vi "Configure Current Limit.vi"(7 "Behavior (0: Regulate)":u16(ring) items=["Regulate", "Trip"], 8 "error in (no error)":errorcluster, 9 "Current Limit (0.0 A)":dbl format="%.3g", 10 "Channel (1: Channel 1)":i32(ring)=1 items=["Channel 1"=1, "Channel 2"=2, "Channel 3"=3], 11 "VISA resource name":refnum<visa-resource-name>) -> (0 "error out":errorcluster, 3 "VISA resource name out":refnum<visa-resource-name>)   [LabVIEW 2020, in "Agilent E363X Series.lvlib"]
doc: "Configures the current limit. Specify the output current limit value and the behavior of the power supply when the output current is greater than or equal to that value."
uses:
  Agilent E363X Series.lvlib
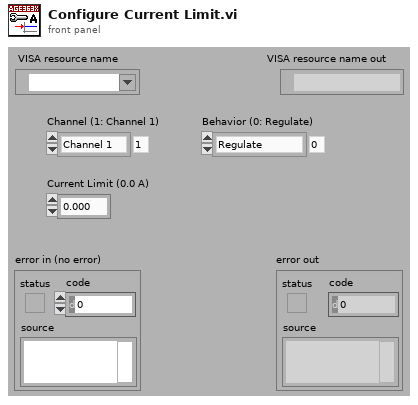
[diagram p1: front panel]
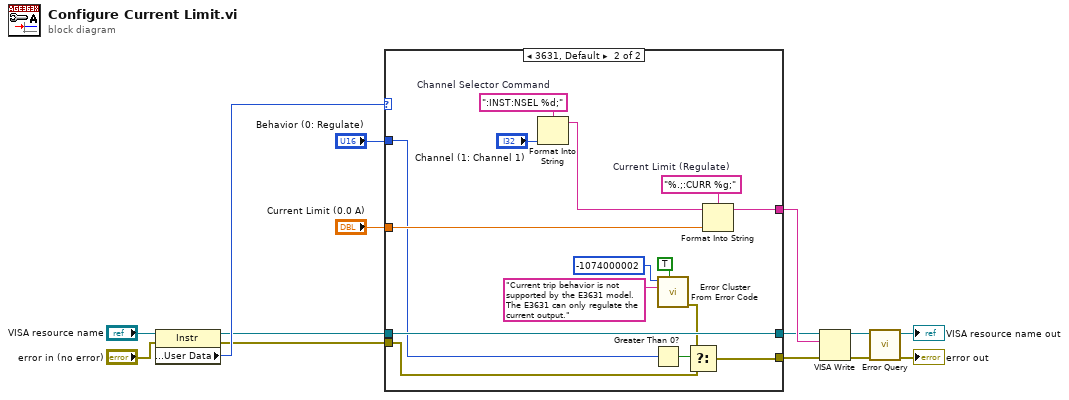
[diagram p0: block diagram]
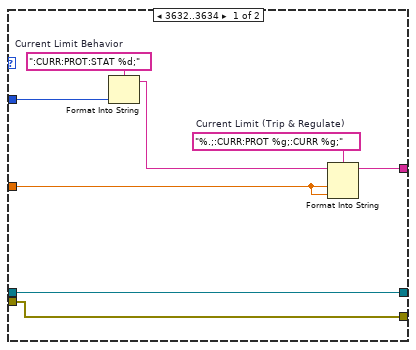
[diagram p2: hidden frame]
diagram:
  n1 = property on="Property Node" class="Instr"(reference="VISA resource name", error in="error in (no error)") -> (reference out=w3:refnum<visa-resource-name>, error out=w4:errorcluster, "General Settings:User Data"=w8:u32)
  n2 = case shown="3631, Default" w8 {
    tunnel: "Behavior (0: Regulate)" -> [w20 w30]
    tunnel: "Current Limit (0.0 A)" -> [w17 w33]
    tunnel: [w19 w32] -> w5
    tunnel: w4 -> [w16 w28]
    tunnel: [w15 w31] -> w2
    tunnel: w3 -> [w15 w31]
    tunnel: [w16 w27] -> w1
    frame 3632..3634 {
      w18 = "%.;:CURR:PROT %g;:CURR %g;"  # Current Limit (Trip & Regulate)
      w22 = ":CURR:PROT:STAT %d;"  # Current Limit Behavior
      n3 = Format Into String(format string=w22, w20) -> (resulting string=w21:string)  [unwired: 2 in, 1 out]
      n4 = Format Into String(format string=w18, initial string=w21, w17, w17) -> (resulting string=w19:string)  [unwired: 1 in, 1 out]
    }
    frame 3631, Default {
      w35 = "%.;:CURR %g;"  # Current Limit (Regulate)
      w37 = ":INST:NSEL %d;"  # Channel Selector Command
      n5 = Format Into String(format string=w37, "Channel (1: Channel 1)") -> (resulting string=w34:string)  [unwired: 2 in, 1 out]
      n6 = Greater Than 0?(x=w30) -> (x > 0?=w29:bool)
      n7 = call <vilib>:"Error Cluster From Error Code.vi"("show call chain? (False)"=TRUE, "error message (\"\")"="Current trip behavior is not supported by the E3631 model.  The E3631 can only regulate the current output." ("error message (\"\")"), "error code (0)"=-1074000002) -> ("error out"=w26:errorcluster)  [unwired: 6 in]
      n8 = Select(t=w26, s=w29, f=w28) -> (s? t:f=w27:errorcluster)
      n9 = Format Into String(format string=w35, initial string=w34, w33) -> (resulting string=w32:string)  [unwired: 1 in, 1 out]
    }
  }
  n10 = VISA Write(VISA resource name=w2, write buffer=w5, error in (no error)=w1) -> (VISA resource name out=w12:refnum<visa-resource-name>, error out=w11:errorcluster)  [unwired: 1 out]
  n11 = call "Error Query.vi"("error in (no error)"=w11, "VISA resource name"=w12) -> ("error out"=→"error out":errorcluster, "VISA resource name out"=→"VISA resource name out":refnum<visa-resource-name>)  [unwired: 6 in, 2 out]
